vi "Compile Engine Init.vi"(8 "error in (no error)":errorcluster, 11 "Device Item Ref in":T2 format="%.0x") -> (0 "error out":errorcluster, 2 "System":T1, 3 "Device Item Ref out":T2 format="%.0x")   [LabVIEW 2015, in "NI 9759 RevB Custom Device.lvlib"]
uses:
  NI 9759 RevB Custom Device.lvlib
  <vilib>/NI Veristand/Custom Device API/Custom Device Item Ref.ctl
  Shared/Types/RT Init Data.ctl
  <vilib>/NI Veristand/Custom Device API/Custom Device Channel Type.ctl
  Shared/9759 Properties.vi
  <vilib>/NI Veristand/Custom Device API/Get Item Property (I32).vi
  <vilib>/NI Veristand/Custom Device API/Get Item Property (String).vi
  <vilib>/NI Veristand/Custom Device API/Get Item Property (Boolean).vi
  <vilib>/NI Veristand/Custom Device API/Get Item Property (Dependent File).vi
  <vilib>/NI VeriStand/Custom Device API/Custom Device API.lvlib
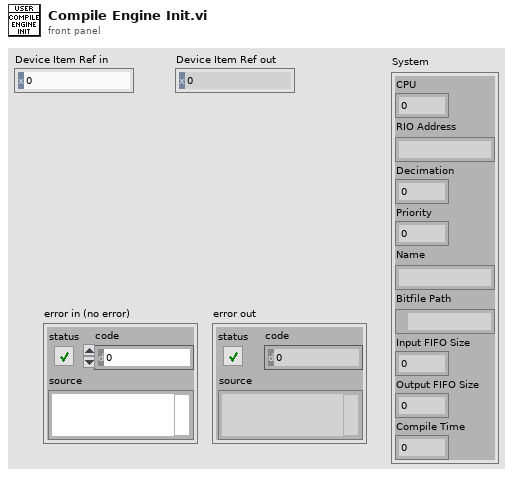
[diagram p1: front panel]
types:
  T1 = typedef "NI 9759 RevB Custom Device.lvlib/RT Init Data.ctl" = cluster{"CPU":i32, "RIO Address":string, "Decimation":i32, "Priority":i32, "Name":string, "Bitfile Path":path, "Input FIFO Size":i32, "Output FIFO Size":i32, "Compile Time":dbl}
  T2 = typedef "Custom Device API.lvlib/Custom Device Item Ref.ctl" = u64
  T3 = typedef "Custom Device API.lvlib/Custom Device Channel Type.ctl" = enum16{"Input", "Output"}
  T4 = typedef "Custom Device API.lvlib/Custom Device Timed Loop Priority.ctl" = enum32{"Low", "Medium", "High"}
  T5 = typedef "Custom Device API.lvlib/Custom Device Item Info.ctl" = cluster{"Name":string, "Is Channel":bool, "GUID":string, "Is Waveform":bool}
  T6 = typedef "Custom Device API.lvlib/Custom Device Target Type.ctl" = enum16{"PharLap", "VxWorks", "Windows"}
  T7 = typedef "Custom Device API.lvlib/Dependent File Optional Info.ctl" = cluster{"Version":string, "RTDestination":path, "ForceDownload":bool, "SupportedTarget":string, "MD5":string}
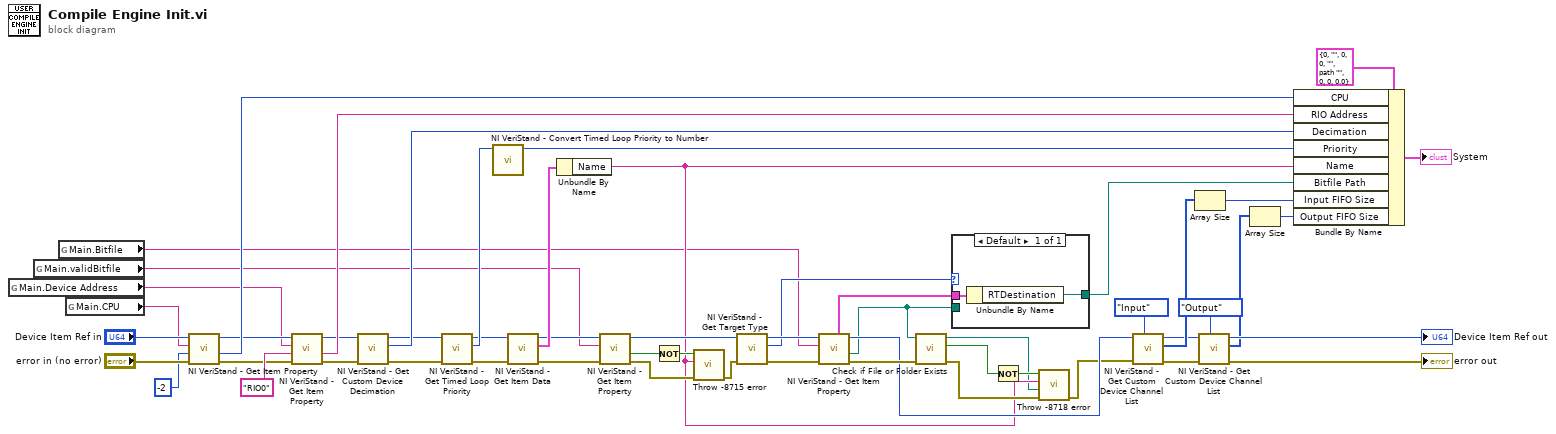
[diagram p0: block diagram]
diagram:
  n1 = global read "9759 Properties.vi" "Main.Device Address"() -> (w2:string)
  n2 = global read "9759 Properties.vi" "Main.validBitfile"() -> (w3:string)
  n3 = global read "9759 Properties.vi" "Main.Bitfile"() -> (w4:string)
  n4 = global read "9759 Properties.vi" "Main.CPU"() -> (w1:string)
  n5 = call-poly <vilib>:"NI VeriStand - Get Item Property.vi"("error in (no error)"="error in (no error)", "Default Value"=-2, "Property Name"=w1, "Item Ref in"="Device Item Ref in") -> ("error out"=w50:errorcluster, "Value"=w53:i32, "Item Ref out"=w51:T2)  [unwired: 4 in, 1 out]
  n6 = call-poly <vilib>:"NI VeriStand - Get Item Property.vi"("error in (no error)"=w50, "Default Value"="RIO0", "Property Name"=w2, "Item Ref in"=w51) -> ("error out"=w49:errorcluster, "Value"=w48:string, "Item Ref out"=w46:T2)  [unwired: 4 in, 1 out]
  n7 = call <vilib>:"NI VeriStand - Get Custom Device Decimation.vi"("error in (no error)"=w49, "Device Ref in"=w46) -> ("error out"=w47:errorcluster, "Decimation"=w45:i32, "Device Ref out"=w43:T2)  [unwired: 7 in]
  n8 = call <vilib>:"NI VeriStand - Get Timed Loop Priority.vi"("error in (no error)"=w47, "Device Ref in"=w43) -> ("error out"=w44:errorcluster, "Priority"=w42:T4, "Device Ref out"=w40:T2)  [unwired: 7 in]
  n9 = call <vilib>:"NI VeriStand - Convert Timed Loop Priority to Number.vi"("Priority"=w42) -> ("Numeric Priority"=w41:i32)  [unwired: 10 in]
  n10 = call <vilib>:"NI VeriStand - Get Item Data.vi"("error in (no error)"=w44, "Item Ref in"=w40) -> ("error out"=w27:errorcluster, "Item Info"=w39:T5, "Item Ref out"=w26:T2)  [unwired: 6 in, 1 out]
  n11 = Unbundle By Name(w39) -> ("Name"=w8:string)
  n12 = call-poly <vilib>:"NI VeriStand - Get Item Property.vi"("error in (no error)"=w27, "Property Name"=w3, "Item Ref in"=w26) -> ("error out"=w32:errorcluster, "Value"=w33:bool, "Item Ref out"=w34:T2)  [unwired: 5 in, 1 out]
  n13 = Not(x=w33) -> (.not. x?=w15:bool)
  n14 = call "Throw -8715 error.vi"("error in (no error)"=w32, "Custom device name"=w8, "Error"=w15) -> ("error out"=w31:errorcluster)  [unwired: 8 in]
  n15 = call <vilib>:"NI VeriStand - Get Target Type.vi"("error in (no error)"=w31, "Item Ref in"=w34) -> ("error out"=w38:errorcluster, "Target Type"=w30:T6, "Item Ref out"=w36:T2)  [unwired: 7 in]
  n16 = call-poly <vilib>:"NI VeriStand - Get Item Property.vi"("error in (no error)"=w38, "Property Name"=w4, "Item Ref in"=w36) -> ("error out"=w37:errorcluster, "Path"=w13:path, "Item Ref out"=w14:T2, "OptionalInfo"=w29:T7)  [unwired: 4 in, 1 out]
  n17 = call <vilib>:"Check if File or Folder Exists.vi"("error in (no error)"=w37, "path"=w13) -> ("error out"=w12:errorcluster, "file or folder exists?"=w10:bool, "dup path"=w7:path)  [unwired: 7 in]
  n18 = case shown="Default" w30 {
    tunnel: w29 -> [w57]
    tunnel: w13 -> [_]
    tunnel: [w56] -> w28
    frame Default {
      n19 = Unbundle By Name(w57) -> ("RTDestination"=w56:path)
    }
  }
  n20 = Not(x=w10) -> (.not. x?=w9:bool)
  n21 = call "Throw -8718 error.vi"("error in (no error)"=w12, "path"=w7, "Custom device name"=w8, "Error"=w9) -> ("error out"=w11:errorcluster)  [unwired: 7 in]
  n22 = call <vilib>:"NI VeriStand - Get Custom Device Channel List.vi"("Channel Type"=Custom_Device_Channel_Type."Input", "error in (no error)"=w11, "Device Ref in"=w14) -> ("error out"=w25:errorcluster, "Specified Channel Ref List"=w23:T2[], "Device Ref out"=w20:T2)  [unwired: 6 in]
  n23 = Array Size(array=w23) -> (size(s)=w22:i32)
  n24 = call <vilib>:"NI VeriStand - Get Custom Device Channel List.vi"("Channel Type"=Custom_Device_Channel_Type."Output", "error in (no error)"=w25, "Device Ref in"=w20) -> ("error out"=→"error out":errorcluster, "Specified Channel Ref List"=w17:T2[], "Device Ref out"=→"Device Item Ref out":T2)  [unwired: 6 in]
  n25 = Array Size(array=w17) -> (size(s)=w16:i32)
  n26 = Bundle By Name(cluster=T1 {"CPU"=0, "RIO Address"="", "Decimation"=0, "Priority"=0, "Name"="", "Bitfile Path"=path "", "Input FIFO Size"=0, "Output FIFO Size"=0, "Compile Time"=0.0} ("System"), "CPU"=w53, "RIO Address"=w48, "Decimation"=w45, "Priority"=w41, "Name"=w8, "Bitfile Path"=w28, "Input FIFO Size"=w22, "Output FIFO Size"=w16) -> (→"System":T1)
